vi "controller_status.vi"(8 "error in (no error)":errorcluster, 11 "VISA Refnum in":refnum<visa-resource-name>) -> (0 "error out":errorcluster, 1 "output cluster":T1, 3 "VISA Refnum out":refnum<visa-resource-name>)   [LabVIEW 2017]
uses:
  Typedefs/Status.ctl
  Typedefs/Error codes.ctl
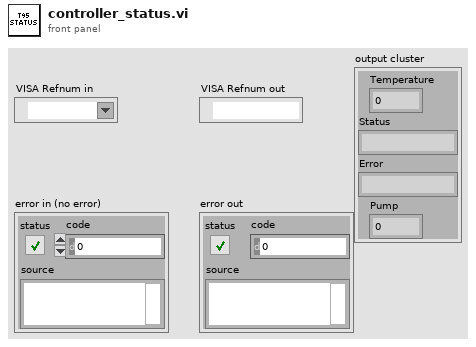
[diagram p1: front panel]
types:
  T1 = cluster{"Temperature":dbl, "Status":string, "Error":string, "Pump":u8}
  T2 = typedef "Status.ctl" = enum16{"No Status", "Stopped", "Heating", "Cooling", "Limit Reached", "Holding the Limit Time", "Manual Hold"}
  T3 = typedef "Error codes.ctl" = enum16{"No Error", "Cooling too fast", "Open Circuit", "Power Surge", "No Exit", "Link Error", ""}
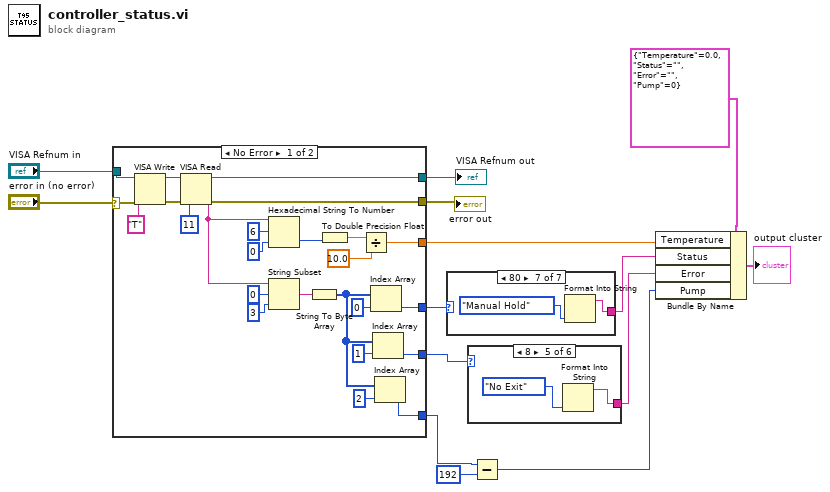
[diagram p0: block diagram]
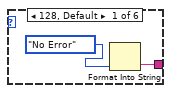
[diagram p2: hidden frame]
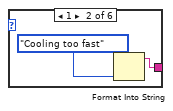
[diagram p3: hidden frame]
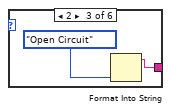
[diagram p4: hidden frame]
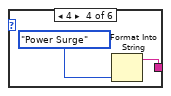
[diagram p5: hidden frame]
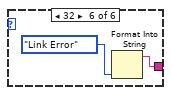
[diagram p6: hidden frame]
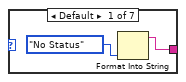
[diagram p7: hidden frame]
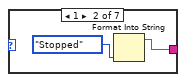
[diagram p8: hidden frame]
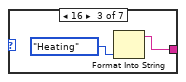
[diagram p9: hidden frame]
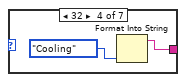
[diagram p10: hidden frame]
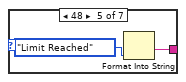
[diagram p11: hidden frame]
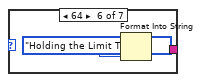
[diagram p12: hidden frame]
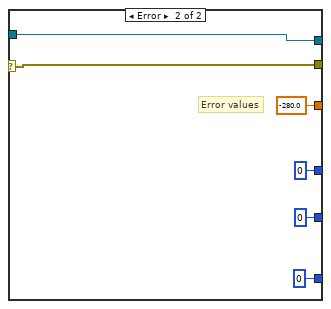
[diagram p13: hidden frame]
diagram:
  n1 = case shown="No Error" "error in (no error)" {
    selector: "error in (no error)" -> [w33 w44]
    tunnel: [w39 w45] -> w14
    tunnel: [w38 w44] -> w13
    tunnel: "VISA Refnum in" -> [w32 w45]
    tunnel: [w21 -280.0] -> w5
    tunnel: [w20 u8 0] -> w10
    tunnel: [w19 u8 0] -> w9
    tunnel: [w15 u8 0] -> w8
    frame No Error {
      n2 = VISA Write(VISA resource name=w32, write buffer="T", error in (no error)=w33) -> (VISA resource name out=w35:refnum<visa-resource-name>, error out=w34:errorcluster)  [unwired: 1 out]
      n3 = VISA Read(VISA resource name=w35, byte count=u32 11, error in (no error)=w34) -> (VISA resource name out=w39:refnum<visa-resource-name>, read buffer=w18:string, error out=w38:errorcluster)  [unwired: 1 out]
      n4 = Hexadecimal String To Number(string=w18, offset=6, default (0uL)=i16 0) -> (number=w22:i16)  [unwired: 1 out]
      n5 = String Subset(string=w18, offset (0)=0, length (rest)=3 ("length (rest)")) -> (substring=w29:string)
      n6 = String To Byte Array(string=w29) -> (unsigned byte array=w17:u8[])
      n7 = To Double Precision Float(number=w22) -> (double precision float=w23:dbl)
      n8 = Divide(x=w23, y=10.0) -> (x/y=w21:dbl)
      n9 = Index Array(array=w17, index=0) -> (element=w20:u8)
      n10 = Index Array(array=w17, index=1) -> (element=w19:u8)
      n11 = Index Array(array=w17, index=2) -> (element=w15:u8)
    }
    frame Error {
      # "Error values"
    }
  }
  "VISA Refnum out" <- w14
  "error out" <- w13
  n12 = case shown="80" w10 {
    tunnel: [w46 w49 w51 w53 w55 w57 w59] -> w4
    frame Default {
      n13 = Format Into String(Status."No Status") -> (resulting string=w46:string)  [unwired: 3 in, 1 out]
    }
    frame 1 {
      n14 = Format Into String(Status."Stopped") -> (resulting string=w49:string)  [unwired: 3 in, 1 out]
    }
    frame 16 {
      n15 = Format Into String(Status."Heating") -> (resulting string=w51:string)  [unwired: 3 in, 1 out]
    }
    frame 32 {
      n16 = Format Into String(Status."Cooling") -> (resulting string=w53:string)  [unwired: 3 in, 1 out]
    }
    frame 48 {
      n17 = Format Into String(Status."Limit Reached") -> (resulting string=w55:string)  [unwired: 3 in, 1 out]
    }
    frame 64 {
      n18 = Format Into String(Status."Holding the Limit Time") -> (resulting string=w57:string)  [unwired: 3 in, 1 out]
    }
    frame 80 {
      n19 = Format Into String(Status."Manual Hold") -> (resulting string=w59:string)  [unwired: 3 in, 1 out]
    }
  }
  n20 = case shown="8" w9 {
    tunnel: [w60 w62 w65 w67 w68 w70] -> w3
    frame 128, Default {
      n21 = Format Into String(Error_codes."No Error") -> (resulting string=w60:string)  [unwired: 3 in, 1 out]
    }
    frame 1 {
      n22 = Format Into String(Error_codes."Cooling too fast") -> (resulting string=w62:string)  [unwired: 3 in, 1 out]
    }
    frame 2 {
      n23 = Format Into String(Error_codes."Open Circuit") -> (resulting string=w65:string)  [unwired: 3 in, 1 out]
    }
    frame 4 {
      n24 = Format Into String(Error_codes."Power Surge") -> (resulting string=w67:string)  [unwired: 3 in, 1 out]
    }
    frame 8 {
      n25 = Format Into String(Error_codes."No Exit") -> (resulting string=w68:string)  [unwired: 3 in, 1 out]
    }
    frame 32 {
      n26 = Format Into String(Error_codes."Link Error") -> (resulting string=w70:string)  [unwired: 3 in, 1 out]
    }
  }
  n27 = Subtract(x=w8, y=u8 192) -> (x-y=w2:u8)
  n28 = Bundle By Name(cluster=T1 {"Temperature"=0.0, "Status"="", "Error"="", "Pump"=0}, "Temperature"=w5, "Status"=w4, "Error"=w3, "Pump"=w2) -> (→"output cluster":T1)
